vi "test_Create Instrument Addon.vi"(8 "error in (no error)":errorcluster, 11 "TestCase in":refnum<class "Instrument Addon Scripting API Custom Device Unit Tests.lvclass">) -> (0 "error out":errorcluster, 3 "TestCase out":refnum<class "Instrument Addon Scripting API Custom Device Unit Tests.lvclass">)   [LabVIEW 2023, in "Instrument Addon Scripting API Custom Device Unit Tests.lvclass"]
uses:
  Instrument Addon Scripting API Custom Device Unit Tests.lvclass
  Includes/Protocols.lvlibp/TCP/TCP Settings.ctl
  Instrument Addon Scripting API Custom Device Unit Tests.lvclass/Instrument Addon Scripting API Custom Device Unit Tests.ctl
  Addon/Addon Shared/SubVIs/Constants.vi
  <vilib>/NI/NI VeriStand Advanced SysDef API/_SubVIs/SysDef.Search.GUID.vi
  NationalInstruments.VeriStand.SystemDefinitionAPI
  <vilib>/addons/_JKI Toolkits/VI Tester/TestCase.llb/TestCase.lvclass
  APIs/Scripting API/Instrument Addon Scripting API.lvlib
  Includes/Protocols.lvlibp/TCP/TCP.lvclass
  <vilib>/NI/NI VeriStand Advanced SysDef API/SysDef API/Advanced System Definition.lvlib
  Addon/Addon Shared/Instrument Addon Shared.lvlib
  Includes/Protocols.lvlibp/Protocol Parent/Protocol Parent.lvclass
  C:/Program Files/National Instruments/LabVIEW 2024/vi.lib/addons/_JKI Toolkits/VI Tester/TestCase.llb/TestCase.lvclass
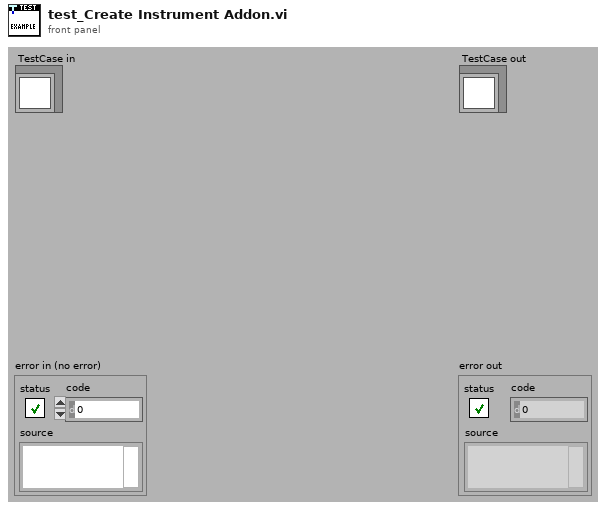
[diagram p1: front panel]
types:
  T1 = typedef "Protocols.lvlibp/TCP.lvclass/TCP Settings.ctl" = cluster{"IP Address":string, "Port":u16}
  T2 = typedef "Custom Device API.lvlib/Custom Device Item Ref.ctl" = u64
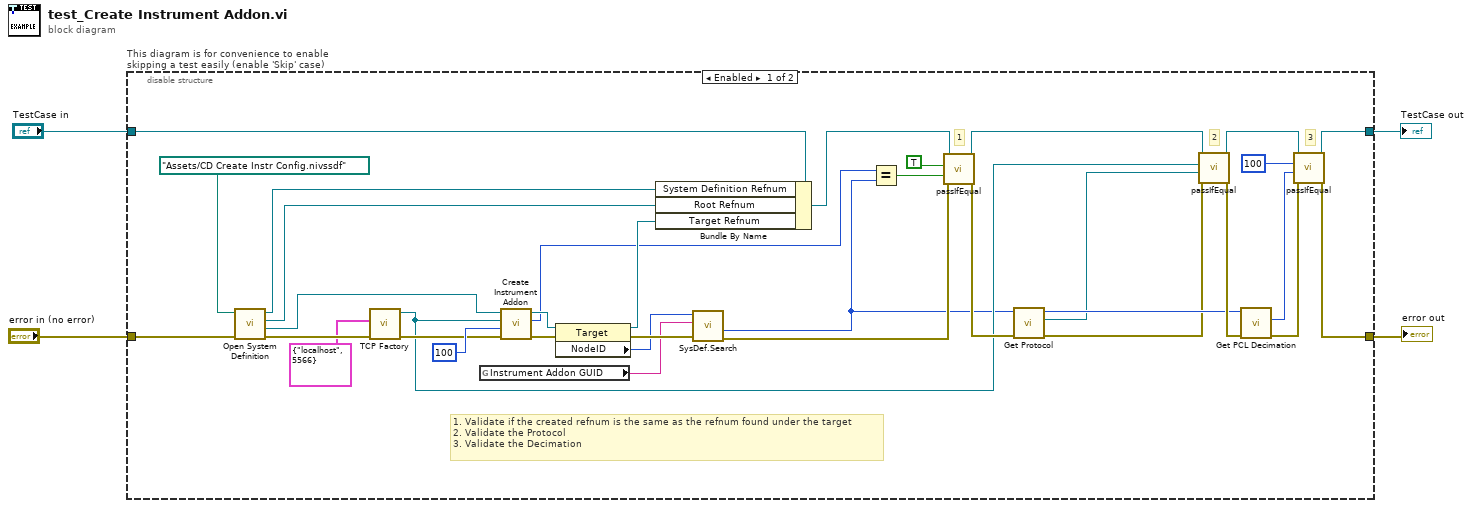
[diagram p0: block diagram]
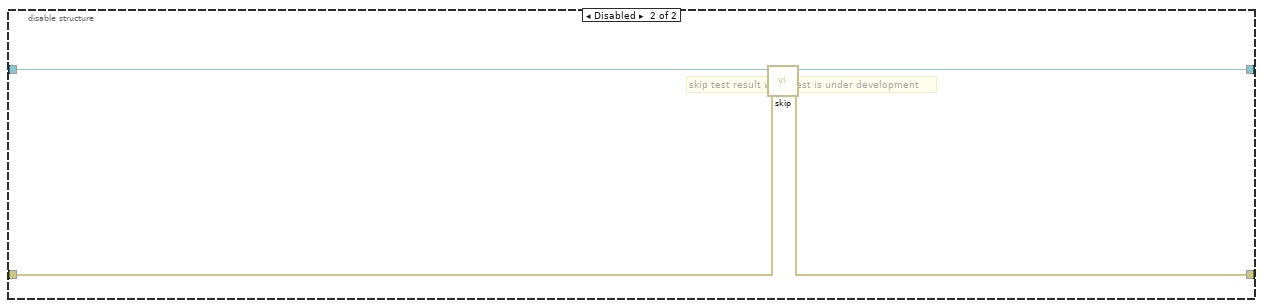
[diagram p2: hidden frame]
diagram:
  n1 = disable-structure "This diagram is for convenience to enable skipping a test easily (enable 'Skip' case)" shown="Enabled" {
    disable-tunnel: "TestCase in" -> [w36 w43]
    disable-tunnel: [w11 w41] -> w1
    disable-tunnel: [w12 w42] -> w3
    disable-tunnel: "error in (no error)" -> [w34 w40]
    frame Enabled {
      # "1. Validate if the created refnum is the same as the refnum found under the target\n2. Validate the Protocol\n3. Validate the Decimation"
      # "3"
      # "2"
      # "1"
      n2 = call "Open System Definition.vi"("error in (no error)"=w34, "System Definition File"=path "Assets/CD Create Instr Config.nivssdf") -> ("error out"=w31:errorcluster, "Target Refnum"=w30:refnum<k24>, "Root Refnum"=w37:refnum<k24>, "System Definition Refnum"=w38:refnum<k24>)  [unwired: 6 in]
      n3 = call "TCP Factory.vi"("error in (no error)"=w31, "TCP settings"=T1 {"IP Address"="localhost", "Port"=5566} ("TCP Settings")) -> ("error out"=w32:errorcluster, "protocol out"=w20:refnum<class "Protocol Parent.lvclass">)  [unwired: 8 in]
      n4 = global read "Constants.vi" "Instrument Addon GUID"() -> (w24:string)
      n5 = call "Create Instrument Addon.vi"("error in (no error)"=w32, "PCL decimation"=u16 100 ("PCL Decimation"), "protocol in"=w20, "target in"=w30) -> ("error out"=w27:errorcluster, "instrument addon refnum"=w9:T2, "target out"=w28:refnum<k24>)  [unwired: 5 in]
      n6 = property class="Target"(reference=w28, error in=w27) -> (reference out=w22:refnum<k24>, error out=w26:errorcluster, "NodeID"=w23:u64)
      n7 = Bundle By Name(cluster=w36, "System Definition Refnum"=w38, "Root Refnum"=w37, "Target Refnum"=w22) -> (w35:refnum<class "Instrument Addon Scripting API Custom Device Unit Tests.lvclass">)
      n8 = call-poly <vilib>:"SysDef.Search.vi"("error in (no error)"=w26, "GUID"=w24, "nodeID"=w23) -> ("error out"=w25:errorcluster, "Value out"=w10:u64)  [unwired: 5 in, 2 out]
      n9 = Equal?(x=w9, y=w10) -> (x = y?=w8:bool)
      n10 = call-dynamic "passIfEqual.vi"("error in (no error)"=w25, "y"=w8, "x"=TRUE ("x = y?"), "TestCase in"=w35) -> ("error out"=w21:errorcluster, "TestCase out"=w19:refnum<class "Instrument Addon Scripting API Custom Device Unit Tests.lvclass">)  [unwired: 6 in]
      n11 = call "Get Protocol.vi"("error in (no error)"=w21, "instrument addon refnum in"=w10) -> ("error out"=w6:errorcluster, "protocol"=w5:refnum<class "Protocol Parent.lvclass">, "instrument addon refnum out"=w17:T2)  [unwired: 7 in]
      n12 = call-dynamic "passIfEqual.vi"("error in (no error)"=w6, "y"=w5, "x"=w20, "TestCase in"=w19) -> ("error out"=w18:errorcluster, "TestCase out"=w13:refnum<class "Instrument Addon Scripting API Custom Device Unit Tests.lvclass">)  [unwired: 6 in]
      n13 = call "Get PCL Decimation.vi"("error in (no error)"=w18, "instrument addon refnum in"=w17) -> ("error out"=w16:errorcluster, "PCL decimation"=w15:u32)  [unwired: 7 in, 1 out]
      n14 = call-dynamic "passIfEqual.vi"("error in (no error)"=w16, "y"=w15, "x"=u32 100 ("PCL Decimation"), "TestCase in"=w13) -> ("error out"=w12:errorcluster, "TestCase out"=w11:refnum<class "Instrument Addon Scripting API Custom Device Unit Tests.lvclass">)  [unwired: 6 in]
    }
    frame Disabled {
      # "skip test result while test is under development"
      n15 = call <vilib>:"skip.vi"("error in (no error)"=w40, "TestCase in"=w43) -> ("error out"=w42:errorcluster, "TestCase out"=w41:refnum<class "Instrument Addon Scripting API Custom Device Unit Tests.lvclass">)  [unwired: 8 in]
    }
  }
  "error out" <- w3
  "TestCase out" <- w1
